vi "Raw_data_to_data.vi"(10 "Trabs precalc":dbl[][](array[numeric]), 11 "Raw data":i32[][][][](array[numeric])) -> (3 "Exp data":dbl[][](graph))   [LabVIEW 2020]
uses:
  average-2Darray-SD_double.vi
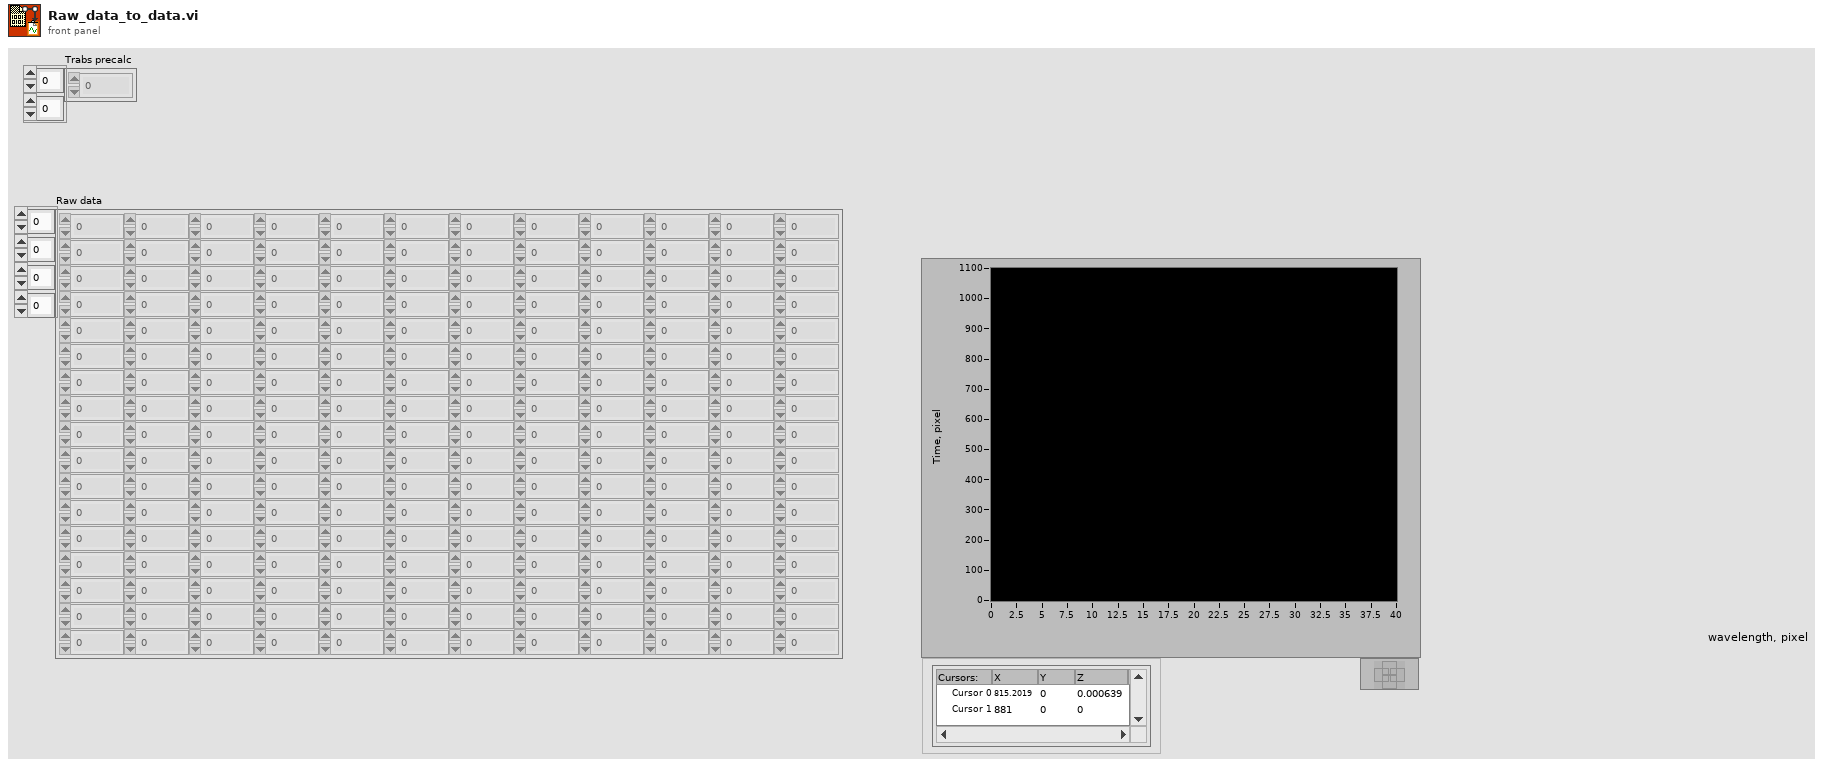
[diagram p1: front panel]
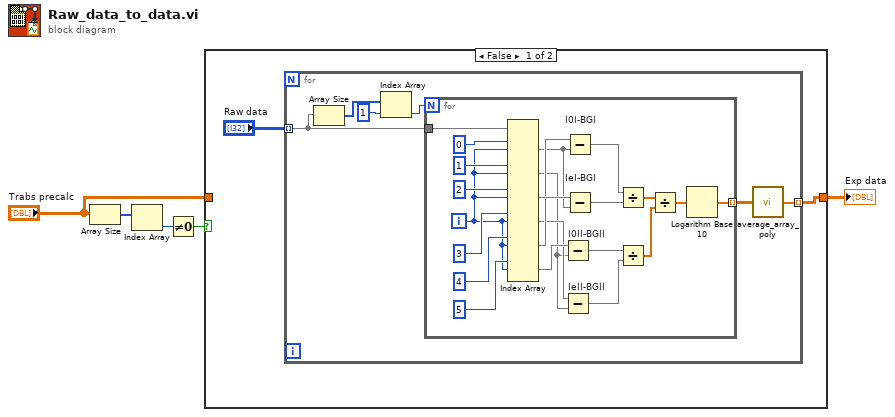
[diagram p0: block diagram]
diagram:
  n1 = Array Size(array="Trabs precalc") -> (size(s)=w4:i32[])
  n2 = Index Array(array=w4) -> (element=w3:i32)  [unwired: 1 in]
  n3 = Not Equal To 0?(x=w3) -> (x != 0?=w2:bool)
  n4 = case shown="False" w2 {
    tunnel: [w6 w36] -> w5
    tunnel: "Trabs precalc" -> [_ w36]
    frame False {
      n5 = for {
        tunnel: "Raw data" -> [w10] mode=indexing
        tunnel: [w8] -> w6 mode=indexing
        n6 = Array Size(array=w10) -> (size(s)=w13:i32[])
        n7 = Index Array(array=w13, index=1) -> (element=w11:i32)
        n8 = for {
          N: w11 -> [_]
          tunnel: w10 -> [w35]
          tunnel: [w18] -> w9 mode=indexing
          i -> [w28]
          n9 = Index Array(array=w35, index (dim 0) #1=0 ("disabled index (page)"), index (dim 1) #1=w28, index (dim 0) #2=1 ("index (page)"), index (dim 1) #2=w28, index (dim 0) #3=2 ("index (page)"), index (dim 1) #3=w28, index (dim 0) #4=3 ("index (page)"), index (dim 1) #4=w28, index (dim 0) #5=4 ("index (page)"), index (dim 1) #5=w28, index (dim 0) #6=5 ("index (page)"), index (dim 1) #6=w28) -> (element #1=w25:i32[], element #2=w22:i32[], element #3=w27:i32[], element #4=w23:i32[], element #5=w26:i32[], element #6=w24:i32[])  [unwired: 6 in]
          n10 = Subtract "I0II-BGII"(x=w24, y=w22) -> (x-y=w15:i32[])
          n11 = Subtract "IeII-BGII"(x=w23, y=w22) -> (x-y=w14:i32[])
          n12 = Subtract "I0I-BGI"(x=w26, y=w25) -> (x-y=w17:i32[])
          n13 = Subtract "IeI-BGI"(x=w27, y=w25) -> (x-y=w16:i32[])
          n14 = Divide(x=w17, y=w16) -> (x/y=w21:dbl[])
          n15 = Divide(x=w15, y=w14) -> (x/y=w20:dbl[])
          n16 = Divide(x=w21, y=w20) -> (x/y=w19:dbl[])
          n17 = Logarithm Base 10(1:w19) -> (0:w18:dbl[])
        }
        n18 = call-poly "average_array_poly.vi"("2D array"=w9) -> ("out array"=w8:dbl[])
      }
    }
    frame True {
    }
  }
  "Exp data" <- w5
